vi "Sequence for Constant Dragging with acquisition bar.vi"() -> ()   [LabVIEW 2012]
doc: "The Sequence VI acquires a sequence of images and displays the images in an image control using high-level acquisition VIs. A sequence is appropriate for applications in which you want to process multiple images."
uses:
  <vilib>/userdefined/High Color/IMAQdx.ctl
  <vilib>/vision/driver/IMAQdx.llb/IMAQdx Acquisition Mode.ctl
  <vilib>/vision/driver/IMAQdx.llb/IMAQdx Buffer Number Mode.ctl
  <vilib>/vision/driver/NI_Vision_Acquisition_Software.lvlib
  <resource>/objmgr/imaqdx.rc
panel:
  in  "Exposure (us)":dbl(slide)=1407.017543859649 min=100.0 max=15000.0 step=100.0 scale=100.0..15000.0
  out "Acquisition  progress":i32(slide) scale=0.0..2999.0
  in  "BitsPerPixel":u32(ring) items=["Use Hardware Value"=0, "10-bit"=10, "12-bit"=12, "14-bit"=14, "16-bit"=16]
  in  "Height":u32=1080
  in  "Width":u32=1920
  in  "Number of Frames":u32=250
  in  "Frame Rate":dbl=55.0
  in  "Path":path
  in  "Camera Name":T1
  out "Image Array":T2[](array[plugin-control])
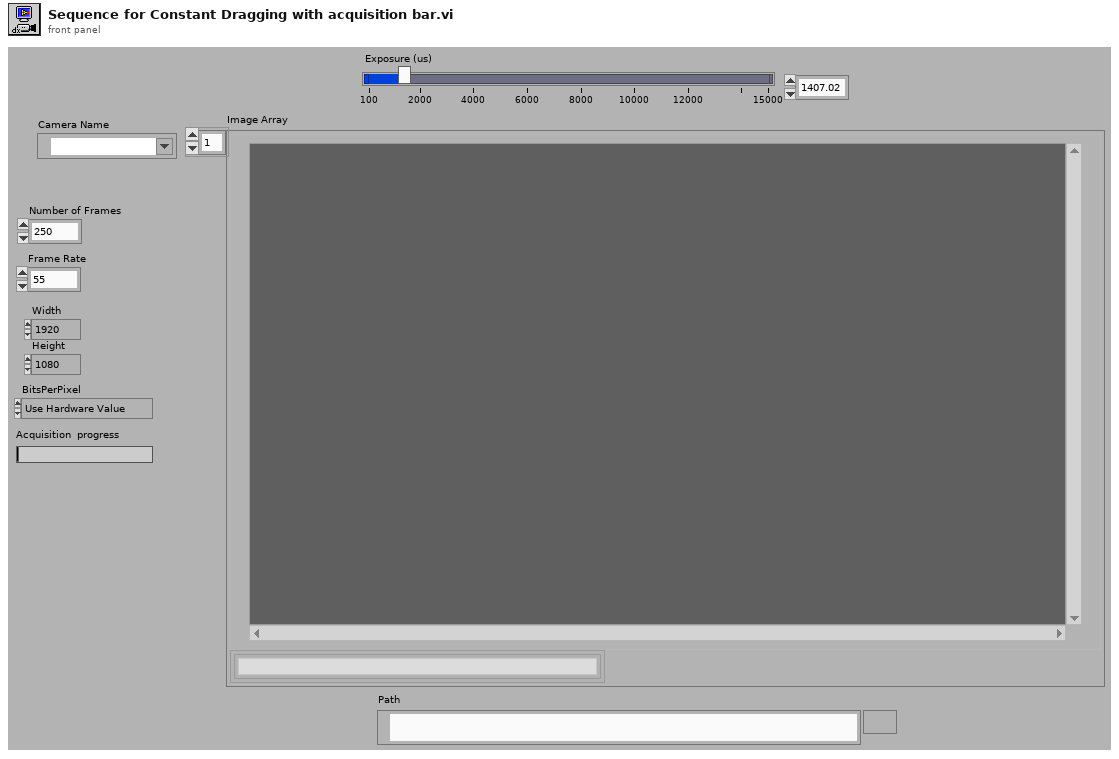
[diagram p1: front panel]
types:
  T1 = typedef "IMAQdx.ctl" = refnum<k21>
  T2 = typedef "IMAQ Image.ctl" = refnum<image>
  T3 = typedef "NI_Vision_Acquisition_Software.lvlib/IMAQdx Acquisition Mode.ctl" = enum32{"One Shot", "Continuous"}
  T4 = typedef "NI_Vision_Acquisition_Software.lvlib/IMAQdx Buffer Number Mode.ctl" = enum32{"Next", "Last", "Buffer Number"}
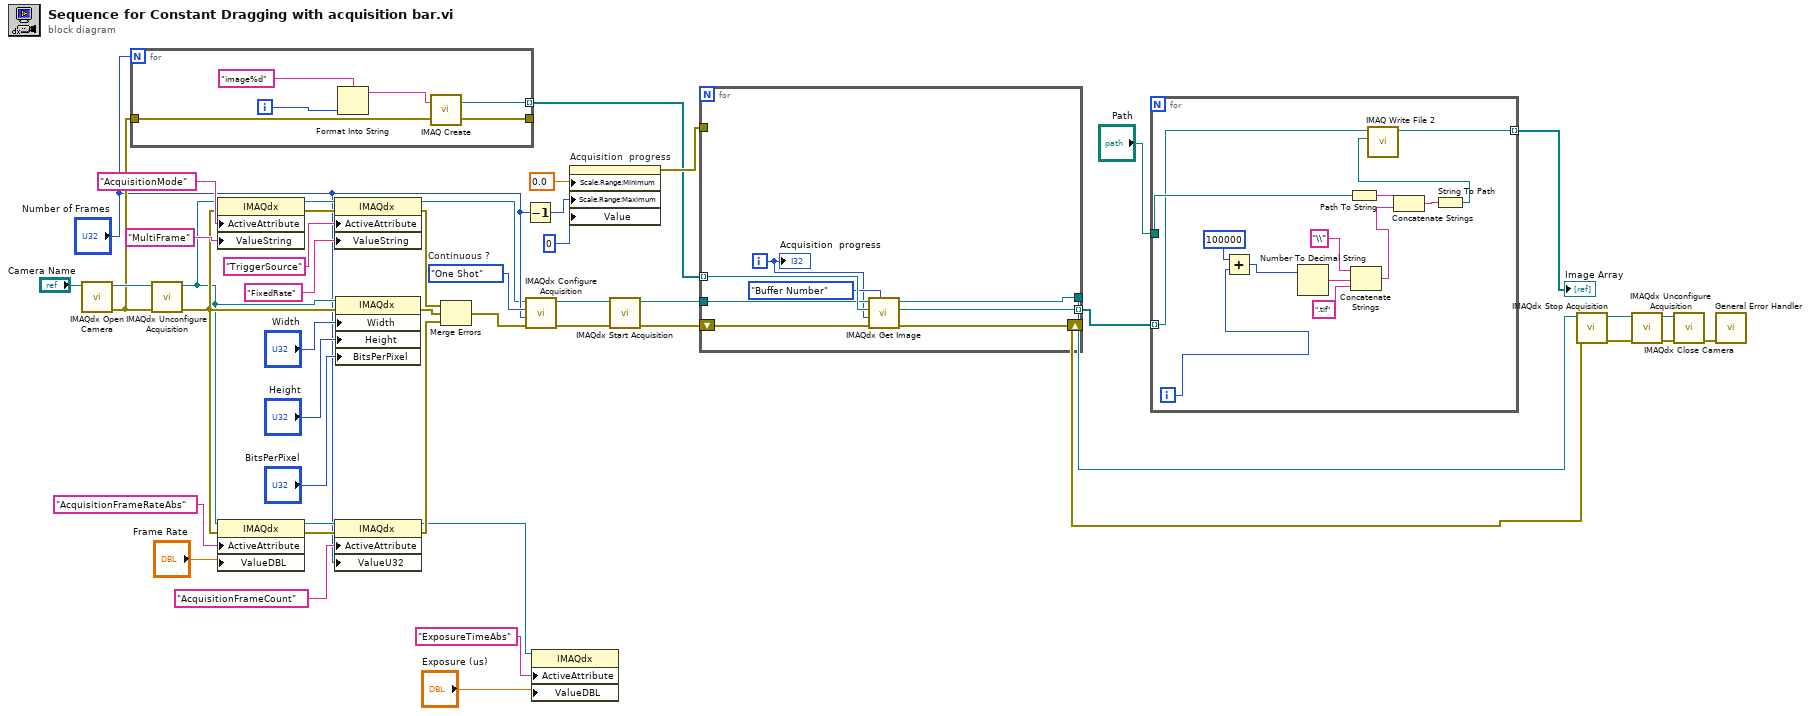
[diagram p0: block diagram]
diagram:
  w25 = IMAQdx_Acquisition_Mode."One Shot"  # Continuous ?
  n1 = call <vilib>:"IMAQdx Open Camera.vi"("Session In"="Camera Name") -> ("error out"=w35:errorcluster, "Session Out"=w36:T1)  [unwired: 2 in, 7 out]
  n2 = for {
    N: "Number of Frames" -> [_]
    tunnel: w35 -> [w54]
    tunnel: [w53] -> w13 mode=indexing
    tunnel: [w52] -> _
    i -> [w51]
    n3 = Format Into String(format string="image%d" ("Image Name"), w51) -> (resulting string=w50:string)  [unwired: 2 in, 1 out]
    n4 = call "IMAQ Create"("Image Name"=w50, "error in (no error)"=w54) -> ("New Image"=w53:T2, "error out"=w52:errorcluster)  [unwired: 2 in, 1 out]
  }
  n5 = call <vilib>:"IMAQdx Unconfigure Acquisition.vi"("error in"=w35, "Session In"=w36) -> ("error out"=w30:errorcluster, "Session Out"=w27:T1)  [unwired: 8 out]
  n6 = property class="IMAQdx"(reference=w27, error in=w30, "ActiveAttribute"="AcquisitionMode", "ValueString"="MultiFrame") -> (reference out=w31:T1, error out=w41:errorcluster)
  n7 = property class="IMAQdx"(reference=w27, error in=w30, "ActiveAttribute"="AcquisitionFrameRateAbs", "ValueDBL"="Frame Rate") -> (reference out=w45:T1, error out=w44:errorcluster)
  n8 = property class="IMAQdx"(reference=w31, error in=w41, "ActiveAttribute"="TriggerSource", "ValueString"="FixedRate") -> (reference out=w11:T1, error out=w37:errorcluster)
  n9 = property class="IMAQdx"(reference=w45, error in=w44, "ActiveAttribute"="AcquisitionFrameCount", "ValueU32"="Number of Frames") -> (reference out=w1:T1, error out=w38:errorcluster)
  n10 = property class="IMAQdx"(reference=w27, error in=w30, "Width"="Width", "Height"="Height", "BitsPerPixel"="BitsPerPixel") -> (error out=w29:errorcluster)  [unwired: 1 out]
  n11 = Merge Errors(w37, w29, w38) -> (w8:errorcluster)
  n12 = Decrement(x="Number of Frames") -> (x-1=w22:u32)
  n13 = call <vilib>:"IMAQdx Configure Acquisition.vi"("error in"=w8, "Number of Buffers"="Number of Frames", "Continuous?"=w25, "Session In"=w11) -> ("error out"=w7:errorcluster, "Session Out"=w10:T1)  [unwired: 6 out]
  n14 = property class="IMAQdx"(reference=w1, "ActiveAttribute"="ExposureTimeAbs", "ValueDBL"="Exposure (us)") -> ()  [unwired: 1 in, 2 out]
  n15 = property on="Acquisition  progress" class="Slide (strict)"("Scale.Range:Minimum"=0.0 ("Write Attribute"), "Scale.Range:Maximum"=w22, "Value"=u32 0 ("Acquisition  progress")) -> (error out=w14:errorcluster)  [unwired: 2 in, 1 out]
  n16 = call <vilib>:"IMAQdx Start Acquisition.vi"("error in"=w7, "Session In"=w10) -> ("error out"=w24:errorcluster, "Session Out"=w9:T1)  [unwired: 8 out]
  n17 = for {
    tunnel: w13 -> [w62] mode=indexing
    shift-right: [w60] -> w21
    shift-left: w24 -> [w61]
    tunnel: [w59] -> w20
    tunnel: w9 -> [w58]
    tunnel: [w55] -> w5 mode=indexing
    tunnel: w14 -> [_]
    i -> [w56]
    n18 = call <vilib>:"IMAQdx Get Image.vi"("Buffer Number Mode (Next)"=IMAQdx_Buffer_Number_Mode."Buffer Number", "error in"=w61, "Buffer Number In"=w56, "Image In"=w62, "Session In"=w58) -> ("error out"=w60:errorcluster, "Image Out"=w55:T2, "Session Out"=w59:T1)  [unwired: 4 out]
    "Acquisition  progress" <- w56
  }
  n19 = for {
    tunnel: "Path" -> [w65]
    tunnel: w5 -> [w64] mode=indexing
    tunnel: [w63] -> w4 mode=indexing
    i -> [w70]
    n20 = Add(x=100000, y=w70) -> (x+y=w72:i32)
    n21 = Number To Decimal String(number=w72) -> (decimal integer string=w75:string)  [unwired: 1 out]
    n22 = Path To String(path=w65) -> (string=w69:string)
    n23 = Concatenate Strings("\\" ("string"), w75, ".tif") -> (w67:string)
    n24 = Concatenate Strings(w69, w67) -> (w68:string)
    n25 = String To Path(string=w68) -> (path=w66:path)
    n26 = call-poly "IMAQ Write File 2"("File Path"=w66, "Image"=w64) -> ("Image Out (duplicate)"=w63:T2)  [unwired: 3 in, 6 out]
  }
  "Image Array" <- w4
  n27 = call <vilib>:"IMAQdx Stop Acquisition.vi"("error in"=w21, "Session In"=w20) -> ("error out"=w19:errorcluster, "Session Out"=w18:T1)  [unwired: 8 out]
  n28 = call <vilib>:"IMAQdx Unconfigure Acquisition.vi"("error in"=w19, "Session In"=w18) -> ("error out"=w17:errorcluster, "Session Out"=w16:T1)  [unwired: 8 out]
  n29 = call <vilib>:"IMAQdx Close Camera.vi"("error in"=w17, "Session In"=w16) -> ("error out"=w26:errorcluster)  [unwired: 9 out]
  n30 = call <vilib>:"General Error Handler.vi"("error in (no error)"=w26) -> ()  [unwired: 1 in, 14 out]
